vi "Get Task ID.vi"(11 "Task in":refnum<class "Task.lvclass">) -> (2 "Task ID":string, 3 "Task out":refnum<class "Task.lvclass">)   [LabVIEW 2020, in "Volatus.lvlib" / "Task.lvclass"]
uses:
  Task.lvclass
  Task.lvclass/Task.ctl
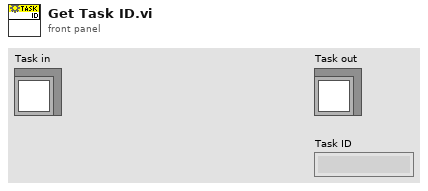
[diagram p1: front panel]
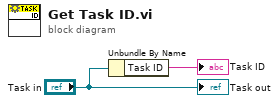
[diagram p0: block diagram]
diagram:
  n1 = Unbundle By Name("Task in") -> ("Task ID"=→"Task ID":string)
  "Task out" <- "Task in"
